vi "Generador de numeros.vi"() -> ()   [LabVIEW 2021]
panel:
  out "error out":errorcluster
  in  "error in (no error)":errorcluster
  in  "stop":bool
  out "Datos Finales":T1(array[cluster])
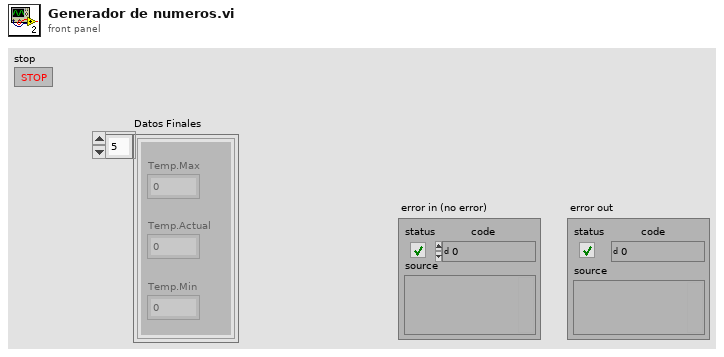
[diagram p1: front panel]
types:
  T1 = cluster{"Temp.Max":dbl, "Temp.Actual":dbl, "Temp.Min":dbl}[]
  T2 = cluster{"number: 0 to 1":dbl, "number: 0 to 1":dbl, "number: 0 to 1":dbl}
  T3 = cluster{"number: 0 to 1":dbl, "number: 0 to 1":dbl, "number: 0 to 1":dbl}[]
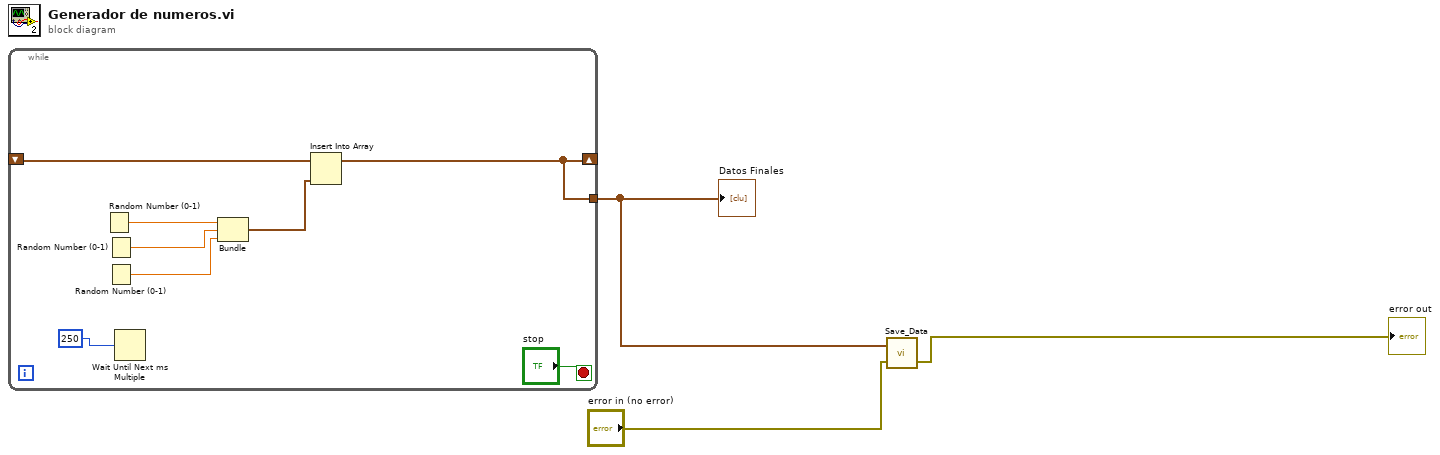
[diagram p0: block diagram]
diagram:
  n1 = while {
    shift-right: [w6] -> _
    shift-left: _ -> [w11]
    tunnel: [w6] -> w3
    stop <- "stop" stop-if-true
    n2 = Random Number (0-1)() -> (number: 0 to 1=w10:dbl)
    n3 = Random Number (0-1)() -> (number: 0 to 1=w9:dbl)
    n4 = Random Number (0-1)() -> (number: 0 to 1=w8:dbl)
    n5 = Wait Until Next ms Multiple(millisecond multiple=u32 250 ("millisecond timer value")) -> ()  [unwired: 1 out]
    n6 = Bundle("number: 0 to 1"=w10, "number: 0 to 1"=w9, "number: 0 to 1"=w8) -> (w7:T2)  [unwired: 1 in]
    n7 = Insert Into Array(array=w11, new element=w7) -> (w6:T3)  [unwired: 1 in]
  }
  "Datos Finales" <- w3
  n8 = call "Save_Data.vi"("error in (no error)"="error in (no error)", "Historial Temperatura"=w3) -> ("error out"=→"error out":errorcluster)  [unwired: 1 in]
